vi "PH_Tektronix_7000.Set Channel Name.vi"(0 "i ref in":refnum<vi>, 1 "Channel":u16(ring) items=["Channel 1", "Channel 2", "Channel 3", "Channel 4", "Math 1", "Math 2", "Math 3", "Math 4", "Reference 1", "Reference 2", "Reference 3", "Reference 4"], 2 "Channel Name":string, 5 "error IO":errorcluster) -> (14 "i ref out":refnum<vi>, 19 "error out":errorcluster)   [LabVIEW 2014, in "PH_Tektronix_7000.lvlib"]
doc: "The incomming Channel Name is written to own attributes and set to the GUI element; afterwards the Channel is configured and the Graph is set."
uses:
  PH_Tektronix_7000.lvlib
  PH_Common/PH_Common.lvlib
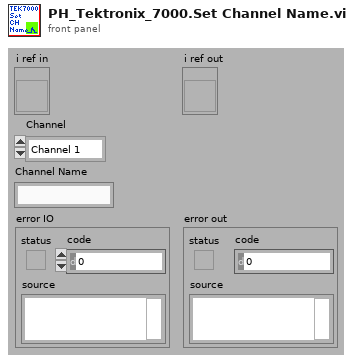
[diagram p1: front panel]
types:
  T1 = typedef "PH_Tektronix_7000.lvlib/PH_Tektronix_7000.i attribute.ctl" = cluster{"VISA Resource Name":refnum<visa-resource-name>, "IDN":cluster{"Instrument Driver":string, "Instrument Firmware":string, "Model":string, "Serial Number":string}, "Selftest":cluster{"Result":i32, "Message":string}, "Trigger Configuration":T2, "Acquisition Configuration":T3, "GUI Refs":T4, "State":T5, "Error Message":string, "Allow Prdc Loop?":bool, "Channel 1":T6, "Channel 2":T6, "Channel 3":T6, "Channel 4":T6, "Data CH 1":waveform(dbl), "Data CH 2":waveform(dbl), "Data CH 3":waveform(dbl), "Data CH 4":waveform(dbl), "Allow config?":bool, "Name Channel 1":string, "Name Channel 2":string, "Name Channel 3":string, "Name Channel 4":string, "Fetch Data before sending to PSDB?":bool, "Constructor passed?":bool, "Data taken at":timestamp, "Plot Colors":u32[], "Default VISA Resource":string}
  T2 = typedef "PH_Tektronix_7000.lvlib/PH_Tektronix_7000.Trigger Config.ctl" = cluster{"Source":u16, "Level [V]":dbl, "Slope":u16, "Coupling":u16, "Trigger Mode":u16}
  T3 = typedef "PH_Tektronix_7000.lvlib/PH_Tektronix_7000.Acquisition Config.ctl" = cluster{"Record Length":u32, "Timebase [s/div]":dbl, "Position [%]":dbl, "Acquisition Type":u16, "Average Waveforms":i32, "Envelope Waveforms":i32, "WfmDB Samples":i32, "Continuous?":bool, "Delay [s]":dbl, "Run?":bool}
  T4 = typedef "PH_Tektronix_7000.lvlib/PH_Tektronix_7000.GUI Refs.ctl" = cluster{"Graph":refnum<vi>, "State":refnum<vi>, "Delete":refnum<vi>, "VISA Resource":refnum<vi>, "Allow Configure":refnum<vi>, "Fetch Data":refnum<vi>, "Fetch before sending Data to PSDB":refnum<vi>, "Name Channel 1":refnum<vi>, "Name Channel 2":refnum<vi>, "Name Channel 3":refnum<vi>, "Name Channel 4":refnum<vi>, "Prdc Intervall [ms]":refnum<vi>, "Data taken":refnum<vi>, "Model":refnum<vi>, "Serial Number":refnum<vi>, "Firmware":refnum<vi>, "Driver":refnum<vi>, "Acquisition":refnum<vi>, "Trigger":refnum<vi>, "Cursor: D Time [s]":refnum<vi>, "Cursor: D Signal [V]":refnum<vi>, "Channel 1":refnum<vi>, "Channel 2":refnum<vi>, "Channel 3":refnum<vi>, "Channel 4":refnum<vi>}
  T5 = typedef "PH_StatusHandler.lvlib/PH_StatusHandler.Status.ctl" = i16
  T6 = typedef "PH_Tektronix_7000.lvlib/PH_Tektronix_7000.Channel Config.ctl" = cluster{"Enable Channel":bool, "Bandwidth":u16, "Input Impedance":u16, "Vertical Coupling":u16, "Probe Attenuation":dbl, "Range [V/div]":dbl, "Position [div]":dbl, "Bandwidth raw":string}
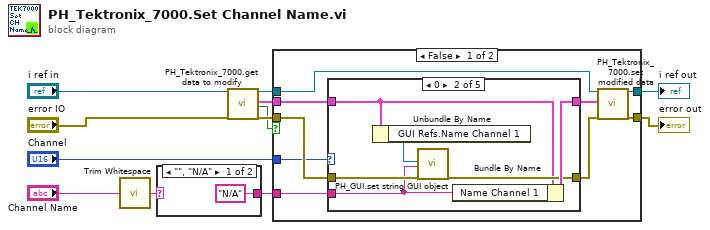
[diagram p0: block diagram]
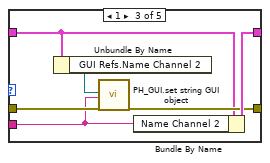
[diagram p4: hidden frame]
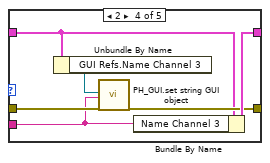
[diagram p5: hidden frame]
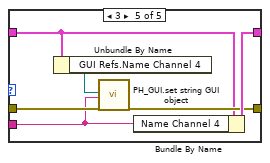
[diagram p6: hidden frame]
diagram:
  n1 = call <vilib>:"Trim Whitespace.vi"("string"="Channel Name") -> ("trimmed string"=w1:string)  [unwired: 1 in]
  n2 = case shown="\"\", \"N/A\"" w1 {
    selector: w1 -> [_ w14]
    tunnel: ["N/A" w14] -> w2
    frame "", "N/A" {
    }
    frame Default {
    }
  }
  n3 = call "PH_Tektronix_7000.get data to modify.vi"("i ref in"="i ref in", "error in (no error)"="error IO") -> ("i ref out"=w8:refnum<vi>, "i attribute"=w6:T1, "timed out"=w7:bool, "error out"=w9:errorcluster)  [unwired: 14 in]
  n4 = case shown="False" w7 {
    tunnel: [w21 w50] -> w4
    tunnel: w9 -> [w20 w50]
    tunnel: w8 -> [w16 w51]
    tunnel: [w22 w51] -> w5
    tunnel: w6 -> [w17 _]
    tunnel: "Channel" -> [w15 _]
    tunnel: w2 -> [w18 _]
    frame False {
      n5 = case shown="0" w15 {
        tunnel: [w25 w31 w37 w43 w49] -> w23
        tunnel: w20 -> [w24 w30 w36 w42 w48]
        tunnel: [w24 w29 w35 w41 w47] -> w19
        tunnel: w18 -> [_ w28 w34 w40 w46]
        tunnel: w17 -> [w25 w27 w33 w39 w45]
        frame Default {
        }
        frame 0 {
          n6 = Unbundle By Name(w27) -> ("GUI Refs.Name Channel 1"=w26:refnum<vi>)
          n7 = call "PH_GUI.set string GUI object.vi"("GUI object Ref"=w26, "Text"=w28, "error in"=w30) -> ("error out"=w29:errorcluster)  [unwired: 16 in]
          n8 = Bundle By Name(cluster=w27, "Name Channel 1"=w28) -> (w31:T1)
        }
        frame 1 {
          n9 = Unbundle By Name(w33) -> ("GUI Refs.Name Channel 2"=w32:refnum<vi>)
          n10 = call "PH_GUI.set string GUI object.vi"("GUI object Ref"=w32, "Text"=w34, "error in"=w36) -> ("error out"=w35:errorcluster)  [unwired: 16 in]
          n11 = Bundle By Name(cluster=w33, "Name Channel 2"=w34) -> (w37:T1)
        }
        frame 2 {
          n12 = Unbundle By Name(w39) -> ("GUI Refs.Name Channel 3"=w38:refnum<vi>)
          n13 = call "PH_GUI.set string GUI object.vi"("GUI object Ref"=w38, "Text"=w40, "error in"=w42) -> ("error out"=w41:errorcluster)  [unwired: 16 in]
          n14 = Bundle By Name(cluster=w39, "Name Channel 3"=w40) -> (w43:T1)
        }
        frame 3 {
          n15 = Unbundle By Name(w45) -> ("GUI Refs.Name Channel 4"=w44:refnum<vi>)
          n16 = call "PH_GUI.set string GUI object.vi"("GUI object Ref"=w44, "Text"=w46, "error in"=w48) -> ("error out"=w47:errorcluster)  [unwired: 16 in]
          n17 = Bundle By Name(cluster=w45, "Name Channel 4"=w46) -> (w49:T1)
        }
      }
      n18 = call "PH_Tektronix_7000.set modified data.vi"("i ref in"=w16, "i attribute"=w23, "error in (no error)"=w19) -> ("i ref out"=w22:refnum<vi>, "error out"=w21:errorcluster)  [unwired: 15 in]
    }
    frame True {
    }
  }
  "i ref out" <- w5
  "error out" <- w4
